vi "Flatten.vi"(8 "error in (no error)":errorcluster, 11 "Analog Out Scan in":refnum<class "Analog Out Scan.lvclass">) -> (0 "error out":errorcluster, 3 "Analog Out Scan out":refnum<class "Analog Out Scan.lvclass">)   [LabVIEW 2017, in "Analog Out Scan.lvclass"]
uses:
  Analog Out Scan.lvclass
  Analog Out Scan.lvclass/Analog Out Scan.ctl
  Global/File Locations.vi
  Scanner/Scanner.lvclass
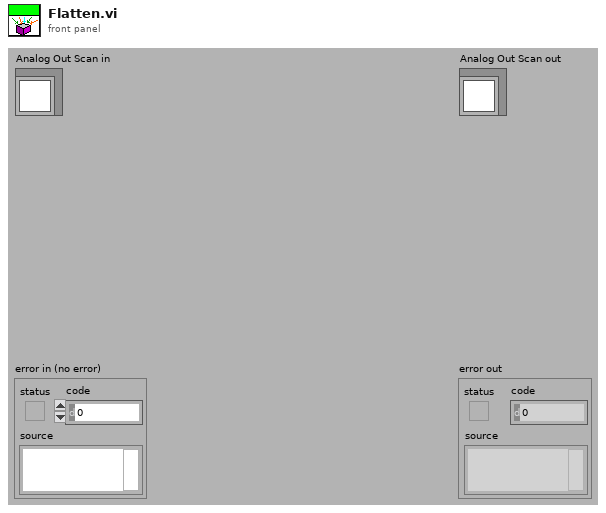
[diagram p1: front panel]
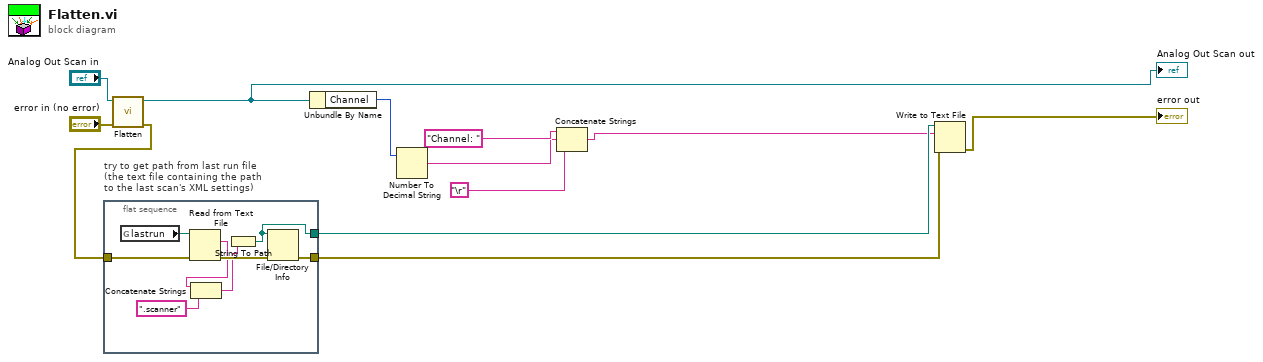
[diagram p0: block diagram]
diagram:
  n1 = flat-sequence "try to get path from last run file\n(the text file containing the path\nto the last scan's XML settings)" {
    tunnel: [w20] -> w8
    tunnel: [w17] -> w7
    tunnel: w10 -> [w16]
    frame #0 {
      n2 = global read "File Locations.vi" "lastrun"() -> (w19:path)
      n3 = Read from Text File(file (use dialog)=w19, error in=w16) -> (text=w15:string, error out=w18:errorcluster)  [unwired: 4 out]
      n4 = Concatenate Strings(w15, ".scanner") -> (w13:string)
      n5 = String To Path(string=w13) -> (path=w20:path)
      n6 = File/Directory Info(path=w20, error in=w18) -> (error out=w17:errorcluster)  [unwired: 6 out]
    }
  }
  n7 = call-parent "Flatten.vi"("error in (no error)"="error in (no error)", "Scanner in"="Analog Out Scan in") -> ("error out"=w10:errorcluster, "Scanner out"=w9:refnum<class "Analog Out Scan.lvclass">)  [unwired: 8 in]
  "Analog Out Scan out" <- w9
  n8 = Unbundle By Name(w9) -> ("Channel"=w3:u8)
  n9 = Number To Decimal String(number=w3) -> (decimal integer string=w4:string)  [unwired: 1 in]
  n10 = Concatenate Strings("Channel: ", w4, "\r") -> (w1:string)
  n11 = Write to Text File(file (use dialog)=w8, text=w1, error in=w7) -> (error out=→"error out":errorcluster)  [unwired: 1 in, 2 out]
